vi "Power Meter Instance.vi"(0 "Power Meter in":refnum<class "Power Meter Base.lvclass">, 5 "Operation":enum16{"Read", "Write", "Clear"}(ring), 11 "error in (no error)":errorcluster) -> (4 "Power Meter out":refnum<class "Power Meter Base.lvclass">, 6 "Found?":bool, 15 "error out":errorcluster)   [LabVIEW 2023, in "RFFixtureCharact.Instruments.lvlib" / "Power Meter Factory.lvclass"]
uses:
  Power Meter Factory.lvclass
  Power Meter Base/Power Meter Base.lvclass
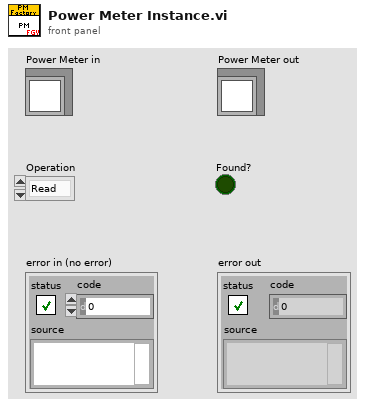
[diagram p1: front panel]
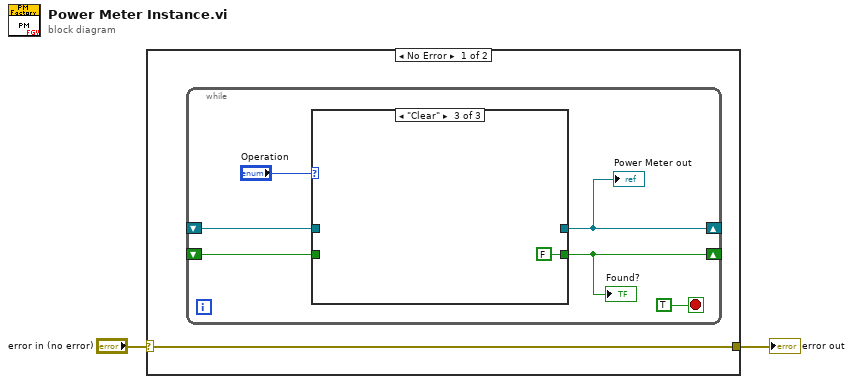
[diagram p0: block diagram]
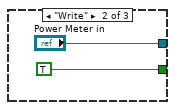
[diagram p3: hidden frame]
diagram:
  n1 = case shown="No Error" "error in (no error)" {
    selector: "error in (no error)" -> [w3 w15]
    tunnel: [w3 w15] -> w2
    frame No Error {
      n2 = while {
        shift-right: [w7] -> _
        shift-left: _ -> [w6]
        shift-right: [w5] -> _
        shift-left: _ -> [w4]
        stop <- TRUE stop-if-true
        n3 = case shown="\"Clear\"" "Operation" {
          tunnel: [w11 "Power Meter in" _] -> w7
          tunnel: w6 -> [w11 _ _]
          tunnel: [w10 TRUE FALSE] -> w5
          tunnel: w4 -> [w10 _ _]
          frame "Read" {
          }
          frame "Write" {
          }
          frame "Clear" {
          }
        }
        "Power Meter out" <- w7
        "Found?" <- w5
      }
    }
    frame Error {
    }
  }
  "error out" <- w2
